vi "Format Duration.vi"(10 "Duration [s]":dbl) -> (2 "String":string)   [LabVIEW 2017, in "Result Tree.lvclass"]
doc: "Returns the text representation for a given duration. The duration is defined in seconds."
uses:
  Result Tree.lvclass
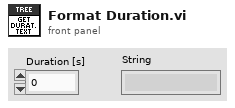
[diagram p1: front panel]
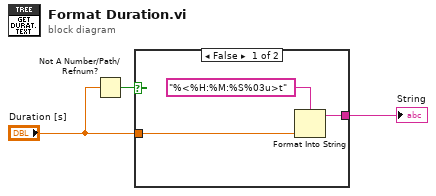
[diagram p0: block diagram]
diagram:
  n1 = Not A Number/Path/Refnum?(number/path/refnum="Duration [s]") -> (NaN/Path/Refnum?=w2:bool)
  n2 = case shown="False" w2 {
    tunnel: "Duration [s]" -> [w4 _]
    tunnel: [w5 _] -> w3
    frame False {
      n3 = Format Into String(format string="%<%H:%M:%S%03u>t", w4) -> (resulting string=w5:string)  [unwired: 2 in, 1 out]
    }
    frame True {
    }
  }
  "String" <- w3
